vi "RichToFlatnixnet_grpc_CanCommResponse.vi"(5 "OutputClusterType":T1, 11 "InputCluster":T4) -> (3 "OutputCluster":T1)   [LabVIEW 2025, in "xnet-grpc_client.lvlib"]
uses:
  nixnet_grpc_CanCommResponse.ctl
  nixnet_grpc_CanCommState.ctl
  nixnet_grpc_CanLastErr.ctl
  nixnet_grpc_CanCommResponse_Flat.ctl
  xnet-grpc_client.lvlib
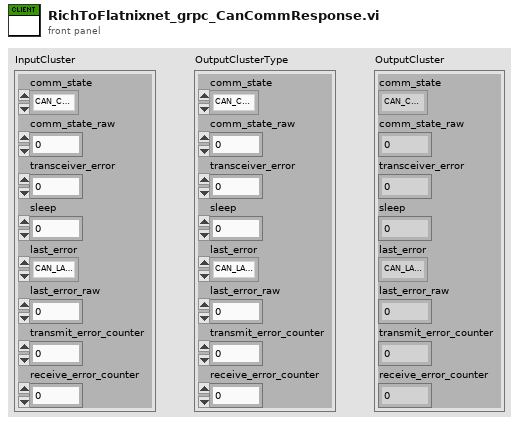
[diagram p1: front panel]
types:
  T1 = typedef "xnet-grpc_client.lvlib/nixnet_grpc_CanCommResponse_Flat.ctl" = cluster{"comm_state":T2, "comm_state_raw":u32, "transceiver_error":u32, "sleep":u32, "last_error":T3, "last_error_raw":u32, "transmit_error_counter":u32, "receive_error_counter":u32}
  T2 = typedef "xnet-grpc_client.lvlib/nixnet_grpc_CanCommState.ctl" = enum32{"CAN_COMM_STATE_ERROR_ACTIVE", "CAN_COMM_STATE_ERROR_PASSIVE", "CAN_COMM_STATE_BUS_OFF", "CAN_COMM_STATE_INIT"}
  T3 = typedef "xnet-grpc_client.lvlib/nixnet_grpc_CanLastErr.ctl" = enum32{"CAN_LAST_ERR_NONE", "CAN_LAST_ERR_STUFF", "CAN_LAST_ERR_FORM", "CAN_LAST_ERR_ACK", "CAN_LAST_ERR_BIT_1", "CAN_LAST_ERR_BIT_0", "CAN_LAST_ERR_CRC"}
  T4 = typedef "xnet-grpc_client.lvlib/nixnet_grpc_CanCommResponse.ctl" = cluster{"comm_state":T2, "comm_state_raw":u32, "transceiver_error":u32, "sleep":u32, "last_error":T3, "last_error_raw":u32, "transmit_error_counter":u32, "receive_error_counter":u32}
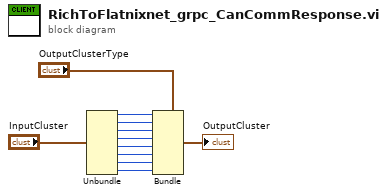
[diagram p0: block diagram]
diagram:
  n1 = Unbundle "Unbundle"("InputCluster") -> ("comm_state"=w8:T2, "comm_state_raw"=w7:u32, "transceiver_error"=w6:u32, "sleep"=w5:u32, "last_error"=w4:T3, "last_error_raw"=w3:u32, "transmit_error_counter"=w2:u32, "receive_error_counter"=w1:u32)
  n2 = Bundle "Bundle"(cluster="OutputClusterType", "comm_state"=w8, "comm_state_raw"=w7, "transceiver_error"=w6, "sleep"=w5, "last_error"=w4, "last_error_raw"=w3, "transmit_error_counter"=w2, "receive_error_counter"=w1) -> (→"OutputCluster":T1)
